vi "LVClass_HasoSlopes Get Slopes X.vi"(0 "HasoSlopes in":refnum<class "HasoSlopes.lvclass">, 11 "error in (no error)":errorcluster) -> (4 "HasoSlopes out":refnum<class "HasoSlopes.lvclass">, 6 "Slopesx":sgl[][](array[numeric]), 15 "error out":errorcluster)   [LabVIEW 2020, in "HasoSlopes.lvclass"]
doc: "HasoSlopes X coordinates getter.\n\n--------------------------------------------------------------------------------\n\n<B>HasoSlopesIn </B> : HasoSlopes object.\n<B>HasoSlopesOut </B> : HasoSlopes object.\n<B>slopes_x </B> : 2D slopes X buffer.\n<B>ErrorIn </B> : Error\n<B>ErrorOut </B> : Error\n\n--------------------------------------------------------------------------------"
uses:
  HasoSlopes.lvclass
  HasoSlopes.lvclass/HasoSlopes.ctl
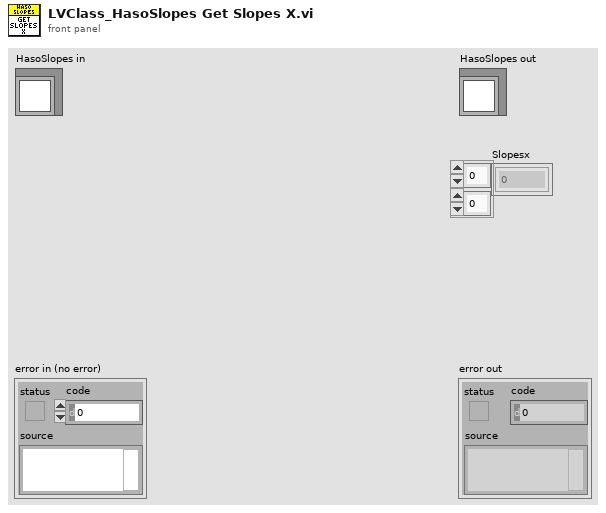
[diagram p1: front panel]
types:
  T1 = typedef "Point2D.ctl" = cluster{"X":u32, "Y":u32}
  T2 = typedef "Point2Df.ctl" = cluster{"X":sgl, "Y":sgl}
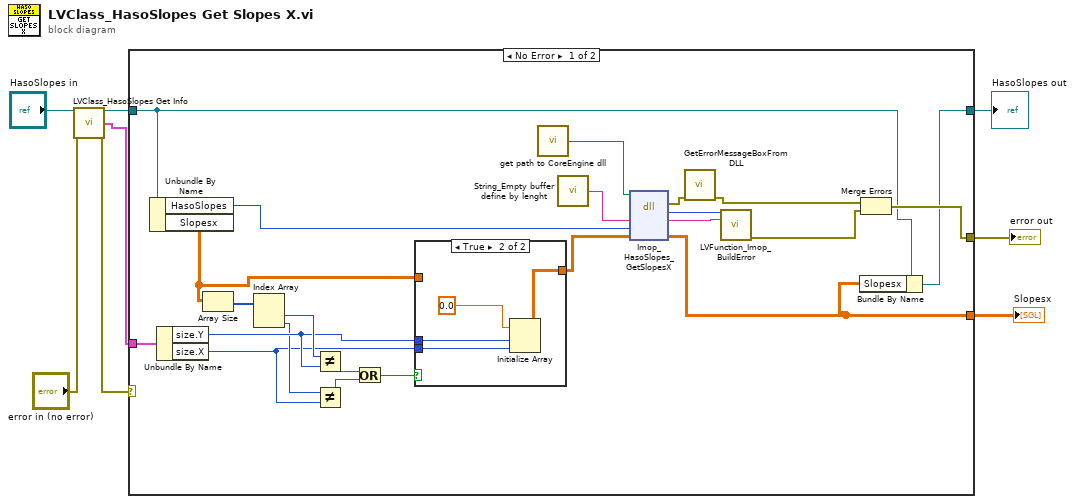
[diagram p0: block diagram]
diagram:
  n1 = call "LVClass_HasoSlopes Get Info.vi"("HasoSlopes in"="HasoSlopes in", "error in (no error)"="error in (no error)") -> ("HasoSlopes out"=w2:refnum<class "HasoSlopes.lvclass">, "dimension"=w1:cluster{"size":T1, "step":T2}, "error out"=w4:errorcluster)  [unwired: 9 in, 2 out]
  n2 = case shown="No Error" w4 {
    selector: w4 -> [_ w38]
    tunnel: [w23 w38] -> w8
    tunnel: [w21 w37] -> w7
    tunnel: w2 -> [w22 w37]
    tunnel: [w9 _] -> w6
    tunnel: w1 -> [w12 _]
    frame No Error {
      n3 = Unbundle By Name(w22) -> ("HasoSlopes"=w28:i32, "Slopesx"=w11:sgl[][])
      n4 = Unbundle By Name(w12) -> ("size.Y"=w18:u32, "size.X"=w16:u32)
      n5 = Array Size(array=w11) -> (size(s)=w20:i32[])
      n6 = Index Array(array=w20) -> (element #1=w19:i32, element #2=w17:i32)  [unwired: 2 in]
      n7 = Not Equal?(x=w19, y=w18) -> (x != y?=w15:bool)
      n8 = Not Equal?(x=w17, y=w16) -> (x != y?=w14:bool)
      n9 = Or(x=w15, y=w14) -> (x .or. y?=w13:bool)
      n10 = case shown="True" w13 {
        tunnel: [w32 w34] -> w10
        tunnel: w18 -> [_ w36]
        tunnel: w16 -> [_ w35]
        tunnel: w11 -> [w32 _]
        frame False {
        }
        frame True {
          n11 = Initialize Array(sgl 0.0, w36, w35) -> (w34:sgl[][])
        }
      }
      n12 = call "get path to CoreEngine dll.vi"() -> ("path to c_interface_vc100.dll"=w27:path)  [unwired: 12 in, 3 out]
      n13 = call "String_Empty buffer define by lenght.vi"() -> ("Empty buffer"=w31:string)  [unwired: 1 in]
      n14 = dll-call lib="D:/soft/HASO_v3/SVN_trunk/ImOpCoreEngine4_LV2011/DLLs/c_interface_vc100.dll" fn="Imop_HasoSlopes_GetSlopesX"(path in=w27, "message"=w31, "objet"=w28, "Slopesx"=w10) -> (error out=w26:errorcluster, "return type"=w29:i32, "message"=w30:string, "Slopesx"=w9:sgl[][])  [unwired: 3 in, 1 out]
      n15 = call "GetErrorMessageBoxFromDLL.vi"("error IN"=w26) -> ("error OUT"=w25:errorcluster)  [unwired: 10 in]
      n16 = call "LVFunction_Imop_BuildError.vi"("code"=w29, "String to Prepend to source (\"\")"=w30) -> ("error out"=w24:errorcluster)  [unwired: 13 in]
      n17 = Bundle By Name(cluster=w22, "Slopesx"=w9) -> (w21:refnum<class "HasoSlopes.lvclass">)
      n18 = Merge Errors(w25, w24) -> (w23:errorcluster)
    }
    frame Error {
    }
  }
  "error out" <- w8
  "HasoSlopes out" <- w7
  "Slopesx" <- w6
